vi "ABB Configure temperatures.vi"() -> ()   [LabVIEW 2017]
uses:
  TC Type.ctl
  RTD Type.ctl
  Temp error msg.ctl
  ABB global.vi
panel:
  in  "Temp error":T1="Error: Temperature measurement "
  in  "RTD Type":T2 items=["PT100 3W", "PT100 4W", "PT1000 3W", "PT1000 4W"]
  out "Readings":dbl[](array[numeric])
  in  "Set RTD name":bool
  in  "thermocouple type":i32(ring)=10072 items=["J"=10072, "K"=10073, "N"=10077, "R"=10082, "S"=10085, "T"=10086, "B"=10047, "E"=10055]
  in  "Thermocouple Type":T3 items=["J", "K", "N", "R", "S", "T", "B", "E"]
  in  "RTDs":i32(listbox)
  in  "Enter Name":T4
  in  "Edit names":T5
  in  "Set TC name":bool
  in  "Thermocouples":i32(listbox)
  in  "Exit":bool
  in  "Temperature names":i32(listbox)
  # "Configure Temperature Measurements"
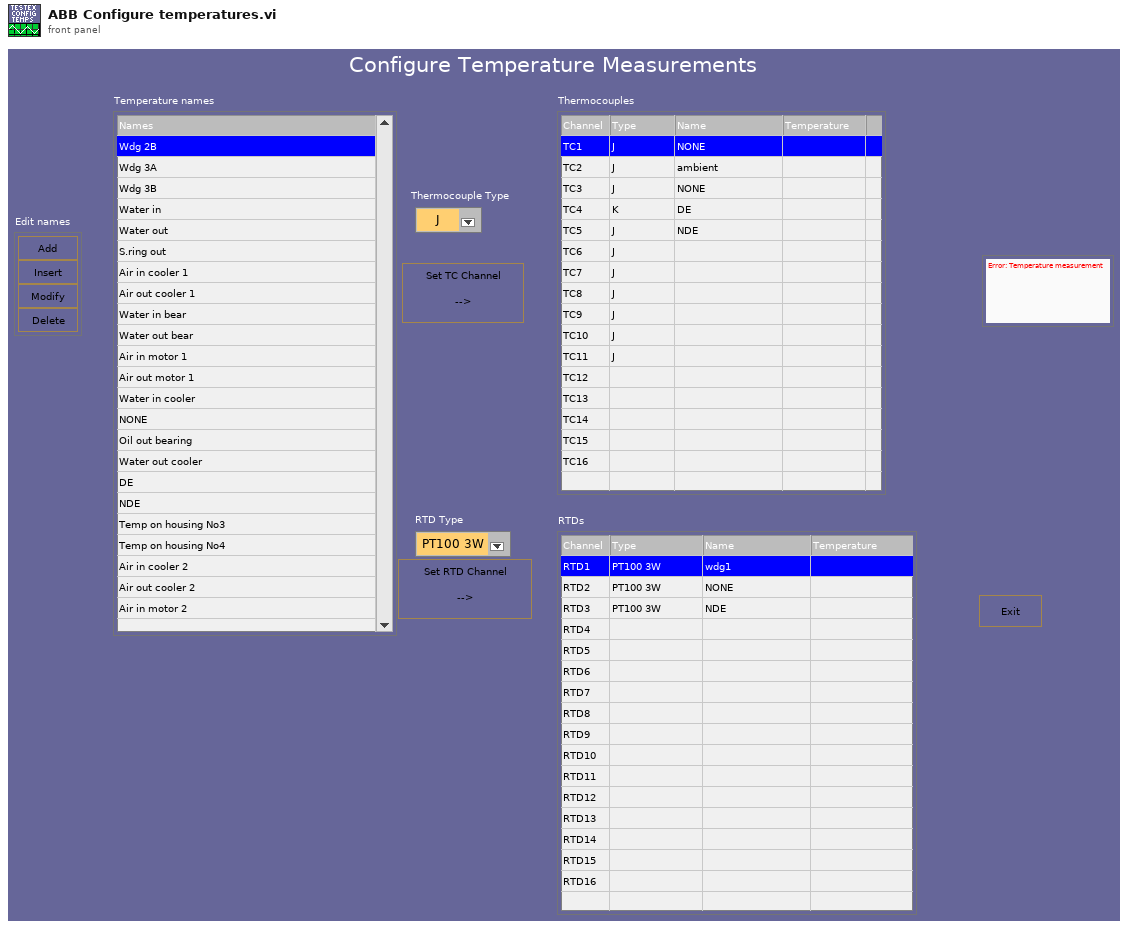
[diagram p1: front panel]
types:
  T1 = typedef "Temp error msg.ctl" = string
  T2 = typedef "RTD Type.ctl" = u16
  T3 = typedef "TC Type.ctl" = u16
  T4 = cluster{"Name":string, "Enter":bool, "Cancel":bool}
  T5 = cluster{"Add":bool, "Insert":bool, "Modify":bool, "Delete":bool}
  T6 = cluster{"Integer":i32, "Dbl":dbl, "String":string, "Boolean":bool}
  T7 = cluster{"Simulate Norma":bool, "Norma 5000 Address":u8, "WebDaq IP Address":string, "Simulate cDAQ":bool}
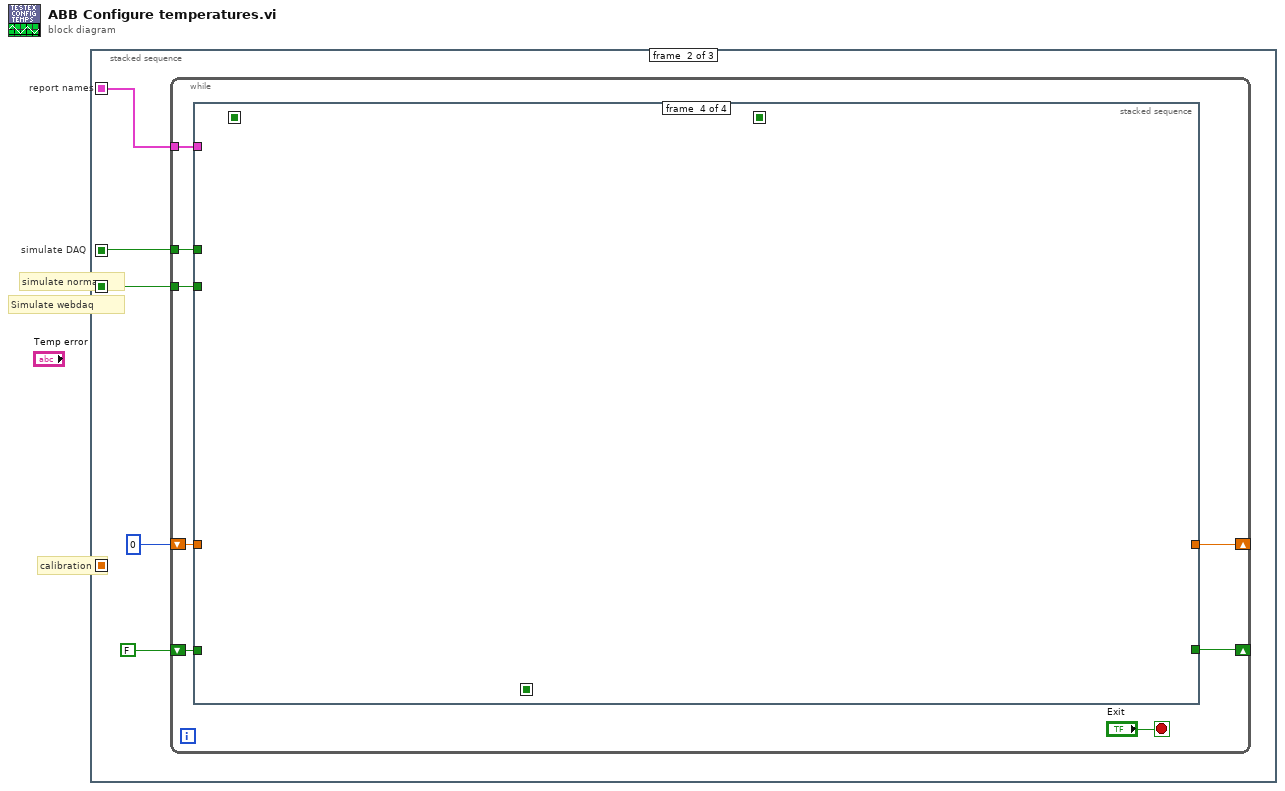
[diagram p0: block diagram]
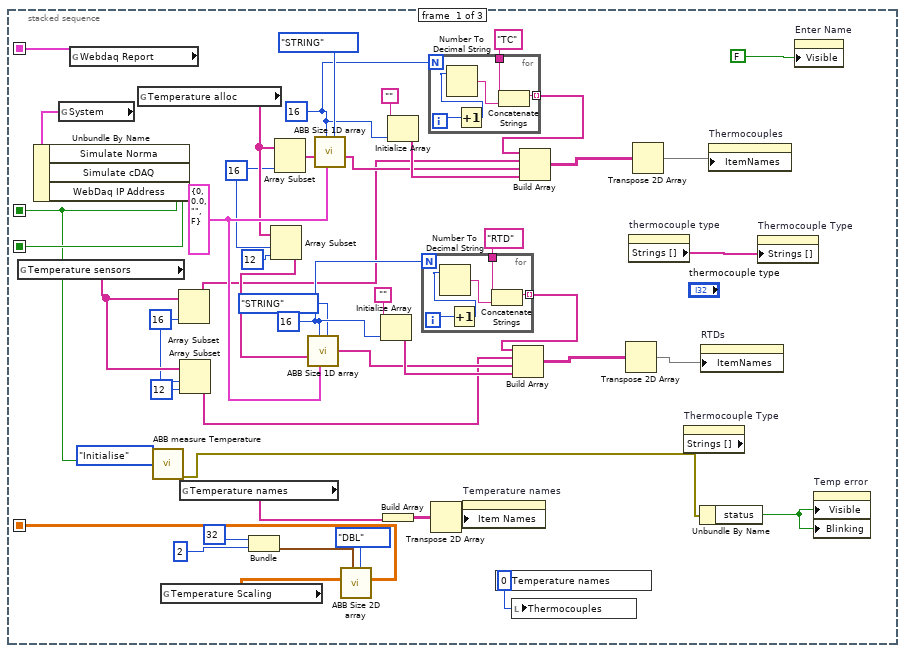
[diagram p2: hidden frame]
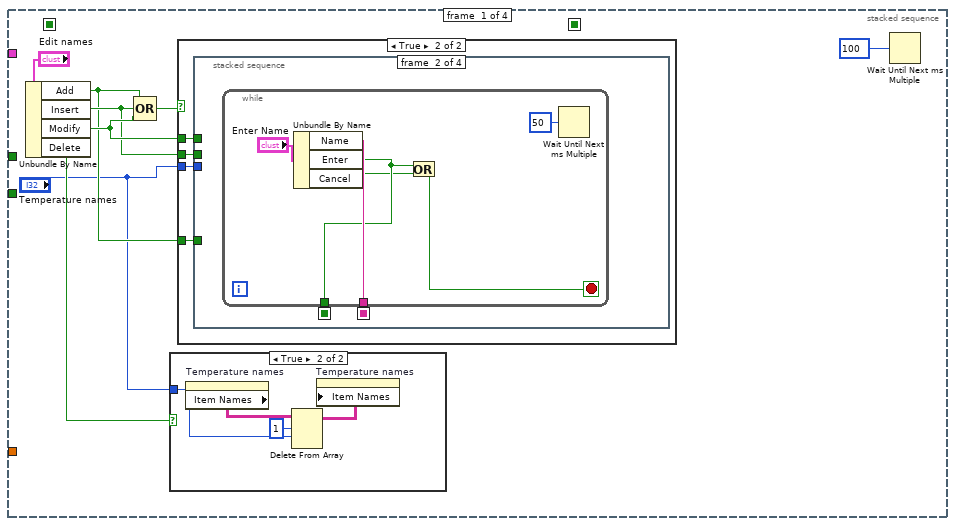
[diagram p3: hidden frame]
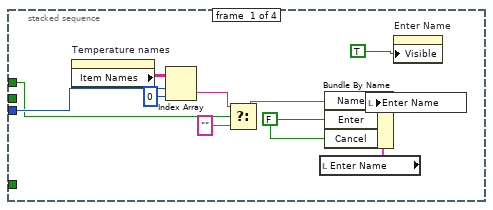
[diagram p6: hidden frame]
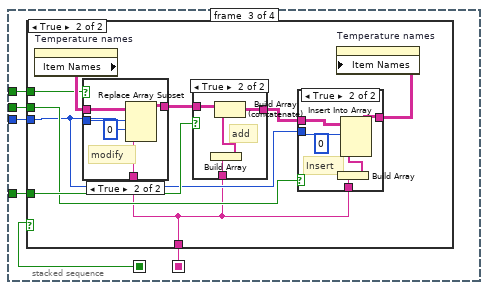
[diagram p7: hidden frame]
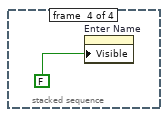
[diagram p12: hidden frame]
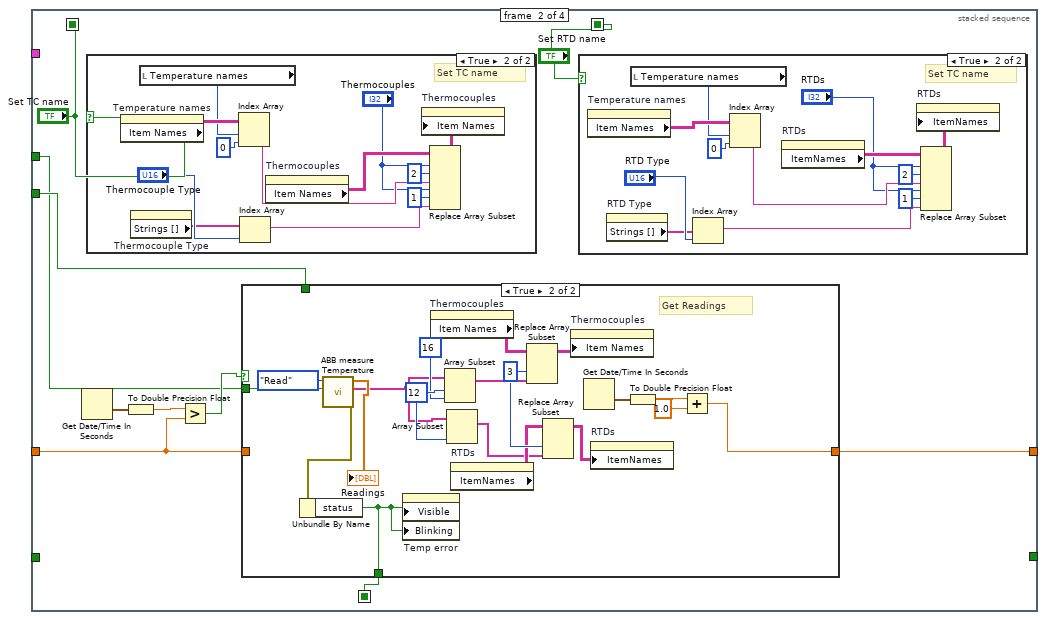
[diagram p13: hidden frame]
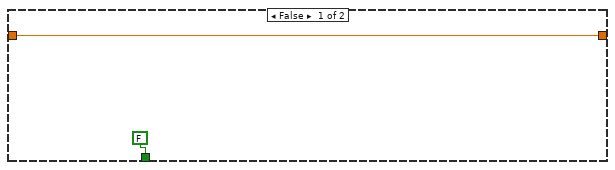
[diagram p15: hidden frame]
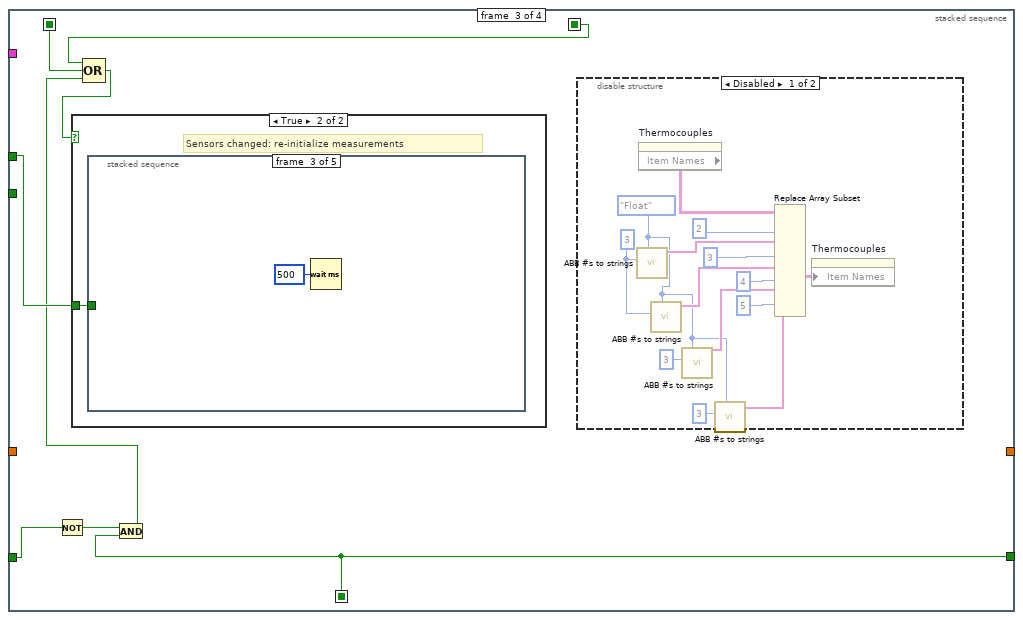
[diagram p17: hidden frame]
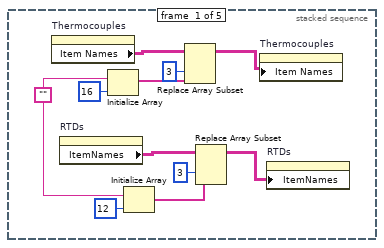
[diagram p20: hidden frame]
diagram:
  # "simulate DAQ"
  # "report names"
  # "Simulate webdaq"
  # "calibration"
  # "simulate norma"
  n1 = stacked-sequence {
    seq-local: [w41 _ _] -> [_ w62 _]
    seq-local: [w35 _ _] -> [_ _ _]
    seq-local: [w33 _ _] -> [_ w61 _]
    seq-local: [w3 _ _] -> [_ w60 w235]
    frame #0 {
      w5 = 16 ("length")
      w17 = 16 ("length")
      w26 = 16 ("Size")
      w20 = T6 {"Integer"=0, "Dbl"=0.0, "String"="", "Boolean"=FALSE} ("Default")
      w43 = 0 ("Temperature names")
      w30 = 16 ("Size")
      n2 = global read "ABB global.vi" "Temperature sensors"() -> (w6:string[])
      n3 = global read "ABB global.vi" "System"() -> (w42:T7)
      n4 = Unbundle By Name(w42) -> ("Simulate Norma"=w41:bool, "Simulate cDAQ"=w3:bool)  [unwired: 1 out]
      n5 = global read "ABB global.vi" "Webdaq Report"() -> (w33:cluster{"Report":string, "Interval":string})
      n6 = global read "ABB global.vi" "Temperature alloc"() -> (w18:string[])
      n7 = call "ABB measure Temperature.vi"("Simulate"=w3, "Mode"=enum16{"Initialise", "Read", "Close"}."Initialise") -> ("error out"=w2:errorcluster)  [unwired: 7 in, 2 out]
      n8 = global read "ABB global.vi" "Temperature Scaling"() -> (w40:dbl[][])
      n9 = Array Subset(array=w6, length=w5) -> (w8:string[])  [unwired: 1 in]
      n10 = Array Subset(array=w6, index=w5, length=12) -> (w4:string[])
      n11 = global read "ABB global.vi" "Temperature names"() -> (w44:string[])
      n12 = Bundle(32, 2) -> (w36:cluster{i32, i32})  [unwired: 1 in]
      n13 = Array Subset(array=w18, index=w17, length=12) -> (w15:string[])
      n14 = Array Subset(array=w18, length=w17) -> (w19:string[])  [unwired: 1 in]
      n15 = call "ABB Size 1D array.vi"("Type"=enum16{"Integer", "DBL", "STRING", "BOOLEAN"}."STRING", "Default"=w20, "Size"=w26, "String Array in"=w15) -> ("String Array out"=w9:string[])  [unwired: 4 in, 3 out]
      n16 = call "ABB Size 1D array.vi"("Type"=enum16{"Integer", "DBL", "STRING", "BOOLEAN"}."STRING", "Default"=w20, "Size"=w30, "String Array in"=w19) -> ("String Array out"=w10:string[])  [unwired: 4 in, 3 out]
      n17 = call "ABB Size 2D array.vi"("Type"=enum16{"Integer", "DBL", "STRING", "BOOLEAN"}."DBL", "Size"=w36, "DBL Array In"=w40) -> ("DBL Array out"=w35:dbl[][])  [unwired: 5 in, 3 out]
      n18 = Initialize Array("", w26) -> (w25:string[])
      n19 = Build Array(w44) -> (w46:string[][])
      n20 = Initialize Array("", w30) -> (w31:string[])
      n21 = for {
        N: w26 -> [_]
        tunnel: "RTD" -> [w53]
        tunnel: [w49] -> w27 mode=indexing
        i -> [w52]
        n22 = Increment(x=w52) -> (x+1=w51:i32)
        n23 = Number To Decimal String(number=w51) -> (decimal integer string=w50:string)  [unwired: 1 in]
        n24 = Concatenate Strings(w53, w50) -> (w49:string)
      }
      n25 = for {
        N: w30 -> [_]
        tunnel: "TC" -> [w58]
        tunnel: [w54] -> w28 mode=indexing
        i -> [w57]
        n26 = Increment(x=w57) -> (x+1=w56:i32)
        n27 = Number To Decimal String(number=w56) -> (decimal integer string=w55:string)  [unwired: 1 in]
        n28 = Concatenate Strings(w58, w55) -> (w54:string)
      }
      n29 = Transpose 2D Array(2D array=w46) -> (transposed array=w45:string[][])
      n30 = property on="Temperature names" class="MCListbox (strict)"("Item Names"=w45) -> ()  [unwired: 2 in, 2 out]
      n31 = local write "Temperature names"(w43) -> ()
      n32 = local write "Thermocouples"(w43) -> ()
      n33 = Build Array(w27, w4, w9, w25) -> (w23:string[][])
      n34 = Build Array(w28, w8, w10, w31) -> (w47:string[][])
      n35 = Transpose 2D Array(2D array=w23) -> (transposed array=w13:string[][])
      n36 = property on="thermocouple type" class="Ring (strict)"() -> ("Strings []"=w12:string[])  [unwired: 2 in, 2 out]
      n37 = Transpose 2D Array(2D array=w47) -> (transposed array=w14:string[][])
      n38 = property on="Thermocouple Type" class="Ring (strict)" props=["Strings []"]() -> ()  [unwired: 2 in, 3 out]
      n39 = Unbundle By Name(w2) -> ("status"=w1:bool)
      n40 = property on="RTDs" class="MCListbox (strict)"("ItemNames"=w13) -> ()  [unwired: 2 in, 2 out]
      n41 = property on="Thermocouples" class="MCListbox (strict)"("ItemNames"=w14) -> ()  [unwired: 2 in, 2 out]
      n42 = property on="Thermocouple Type" class="Ring (strict)"("Strings []"=w12) -> ()  [unwired: 2 in, 2 out]
      n43 = property on="Enter Name" class="Clust (strict)"("Visible"=FALSE) -> ()  [unwired: 2 in, 2 out]
      n44 = property on="Temp error" class="Str (strict)"("Visible"=w1, "Blinking"=w1) -> ()  [unwired: 2 in, 2 out]
    }
    frame #1 {
      n45 = while {
        shift-right: [w69] -> _
        shift-left: 0 -> [w70]
        tunnel: w62 -> [w68]
        tunnel: w61 -> [w67]
        tunnel: w60 -> [w66]
        shift-right: [w65] -> _
        shift-left: FALSE ("status") -> [w64]
        stop <- "Exit" stop-if-true
        n46 = stacked-sequence {
          seq-local: [_ "Set TC name" _ _] -> [_ _ w202 _]
          seq-local: [_ "Set RTD name" _ _] -> [_ _ w201 _]
          seq-local: [_ w140 _ _] -> [_ _ w198 _]
          tunnel: w70 -> [_ w147 _ _]
          tunnel: [_ w149 _ _] -> w69
          tunnel: w68 -> [_ w144 _ _]
          tunnel: w67 -> [_ _ _ _]
          tunnel: w66 -> [_ w141 w199 _]
          tunnel: [_ _ w198 _] -> w65
          tunnel: w64 -> [_ _ w197 _]
          frame #0 {
            n47 = Unbundle By Name("Edit names") -> ("Add"=w74:bool, "Insert"=w75:bool, "Modify"=w76:bool, "Delete"=w73:bool)
            n48 = Compound Arithmetic op=OR(w74, w75, w76) -> (w77:bool)
            n49 = case shown="True" w73 {
              tunnel: "Temperature names" -> [_ w83]
              frame False {
              }
              frame True {
                n50 = property on="Temperature names" class="MCListbox (strict)"() -> ("Item Names"=w82:string[][])  [unwired: 2 in, 2 out]
                n51 = Delete From Array(array=w82, length=1, index (row)=w83) -> (array with subset deleted=w81:string[][])  [unwired: 1 in, 1 out]
                n52 = property on="Temperature names" class="MCListbox (strict)"("Item Names"=w81) -> ()  [unwired: 2 in, 2 out]
              }
            }
            n53 = case shown="True" w77 {
              tunnel: w76 -> [_ w87]
              tunnel: "Temperature names" -> [_ w86]
              tunnel: w75 -> [_ w85]
              tunnel: w74 -> [_ w84]
              frame False {
              }
              frame True {
                n54 = stacked-sequence {
                  seq-local: [_ w100 _ _] -> [_ _ w108 _]
                  seq-local: [_ w99 _ _] -> [_ _ w109 _]
                  tunnel: w87 -> [w95 _ w112 _]
                  tunnel: w86 -> [w98 _ w110 _]
                  tunnel: w85 -> [_ _ w111 _]
                  tunnel: w84 -> [_ _ w107 _]
                  frame #0 {
                    w89 = FALSE ("Enter")
                    n55 = property on="Temperature names" class="MCListbox (strict)"() -> ("Item Names"=w97:string[][])  [unwired: 2 in, 2 out]
                    n56 = Index Array(array=w97, index (row)=w98, index (col)=0 ("disabled index (col)")) -> (element=w94:string)
                    n57 = Select(t=w94, s=w95, f="") -> (s? t:f=w90:string)
                    n58 = local read "Enter Name"() -> (w92:T4)
                    n59 = Bundle By Name(cluster=w92, "Name"=w90, "Enter"=w89, "Cancel"=w89) -> (w91:T4)
                    n60 = local write "Enter Name"(w91) -> ()
                    n61 = property on="Enter Name" class="Clust (strict)"("Visible"=TRUE) -> ()  [unwired: 2 in, 2 out]
                  }
                  frame #1 {
                    n62 = while {
                      tunnel: [w104] -> w100
                      tunnel: [w103] -> w99
                      stop <- w101 stop-if-true
                      n63 = Unbundle By Name("Enter Name") -> ("Name"=w104:string, "Enter"=w103:bool, "Cancel"=w102:bool)
                      n64 = Or(x=w103, y=w102) -> (x .or. y?=w101:bool)
                      n65 = Wait Until Next ms Multiple(millisecond multiple=u32 50) -> ()  [unwired: 1 out]
                    }
                  }
                  frame #2 {
                    n66 = case shown="True" w109 {
                      tunnel: w112 -> [_ w120]
                      tunnel: w111 -> [_ w116]
                      tunnel: w110 -> [_ w115]
                      tunnel: w108 -> [_ w113]
                      tunnel: w107 -> [_ w117]
                      frame False {
                      }
                      frame True {
                        n67 = property on="Temperature names" class="MCListbox (strict)"() -> ("Item Names"=w121:string[][])  [unwired: 2 in, 2 out]
                        n68 = case shown="True" w120 {
                          tunnel: w121 -> [w133 w138]
                          tunnel: [w133 w137] -> w119
                          tunnel: w115 -> [_ w136]
                          tunnel: w113 -> [_ w134]
                          frame False {
                          }
                          frame True {
                            # "modify"
                            n69 = Replace Array Subset(array=w138, new element=w134, index (row)=w136, index (col)=0 ("disabled index (col)")) -> (w137:string[][])
                          }
                        }
                        n70 = case shown="True" w117 {
                          tunnel: w119 -> [w128 w132]
                          tunnel: w113 -> [_ w131]
                          tunnel: [w128 w129] -> w118
                          frame False {
                          }
                          frame True {
                            # "add"
                            n71 = Build Array(w131) -> (w130:string[])
                            n72 = Build Array (concatenate)(w132, w130) -> (w129:string[][])
                          }
                        }
                        n73 = case shown="True" w116 {
                          tunnel: w118 -> [w122 w127]
                          tunnel: [w122 w126] -> w114
                          tunnel: w115 -> [_ w125]
                          tunnel: w113 -> [_ w124]
                          frame False {
                          }
                          frame True {
                            (unwired) 0 ("disabled index (col)")
                            # "Insert"
                            n74 = Build Array(w124) -> (w123:string[])
                            n75 = Insert Into Array(array=w127, index (row)=w125, new element=w123) -> (w126:string[][])  [unwired: 1 in]
                          }
                        }
                        n76 = property on="Temperature names" class="MCListbox (strict)"("Item Names"=w114) -> ()  [unwired: 2 in, 2 out]
                      }
                    }
                  }
                  frame #3 {
                    n77 = property on="Enter Name" class="Clust (strict)"("Visible"=FALSE) -> ()  [unwired: 2 in, 2 out]
                  }
                }
              }
            }
            n78 = Wait Until Next ms Multiple(millisecond multiple=u32 100) -> ()  [unwired: 1 out]
          }
          frame #1 {
            n79 = Get Date/Time In Seconds() -> (seconds since 1Jan1904=w148:timestamp)
            n80 = case shown="True" "Set TC name" {
              frame False {
              }
              frame True {
                # "Set TC name"
                n81 = property on="Temperature names" class="MCListbox (strict)"() -> ("Item Names"=w194:string[][])  [unwired: 2 in, 2 out]
                n82 = property on="Thermocouple Type" class="Ring (strict)"() -> ("Strings []"=w184:string[])  [unwired: 2 in, 2 out]
                n83 = local read "Temperature names"() -> (w193:i32)
                n84 = Index Array(array=w194, index (row)=w193, index (col)=0 ("disabled index (col)")) -> (element=w189:string)
                n85 = Index Array(array=w184, index="Thermocouple Type") -> (element=w185:string)
                n86 = property on="Thermocouples" class="MCListbox (strict)"() -> ("Item Names"=w191:string[][])  [unwired: 2 in, 2 out]
                n87 = Replace Array Subset(array=w191, new element #1=w189, index (row) #1="Thermocouples", index (col) #1=2 ("disabled index (col)"), new element #2=w185, index (row) #2="Thermocouples", index (col) #2=1 ("disabled index (col)")) -> (w188:string[][])
                n88 = property on="Thermocouples" class="MCListbox (strict)"("Item Names"=w188) -> ()  [unwired: 2 in, 2 out]
              }
            }
            n89 = To Double Precision Float(number=w148) -> (double precision float=w145:dbl)
            n90 = Greater?(x=w145, y=w147) -> (0:w146:bool)
            n91 = case shown="True" w146 {
              tunnel: w147 -> [w163 _]
              tunnel: [w163 w177] -> w149
              tunnel: w144 -> [_ _]
              tunnel: w141 -> [_ w167]
              tunnel: [FALSE ("status") w165] -> w140
              frame False {
              }
              frame True {
                w174 = 12 ("index")
                w173 = 3 ("disabled index (col)")
                # "Get Readings"
                n92 = call "ABB measure Temperature.vi"("Simulate"=w167, "Mode"=enum16{"Initialise", "Read", "Close"}."Read") -> ("error out"=w166:errorcluster, "Reading strings"=w164:string[], "Readings"=→"Readings":dbl[])  [unwired: 7 in]
                n93 = Unbundle By Name(w166) -> ("status"=w165:bool)
                n94 = property on="Temp error" class="Str (strict)"("Visible"=w165, "Blinking"=w165) -> ()  [unwired: 2 in, 2 out]
                n95 = property on="Thermocouples" class="MCListbox (strict)"() -> ("Item Names"=w182:string[][])  [unwired: 2 in, 2 out]
                n96 = Array Subset(array=w164, index=w174, length=16) -> (w175:string[])
                n97 = Array Subset(array=w164, length=w174) -> (w170:string[])  [unwired: 1 in]
                n98 = property on="RTDs" class="MCListbox (strict)"() -> ("ItemNames"=w172:string[][])  [unwired: 2 in, 2 out]
                n99 = Replace Array Subset(array=w182, new element=w175, index (col)=w173) -> (w181:string[][])  [unwired: 1 in]
                n100 = Replace Array Subset(array=w172, new element=w170, index (col)=w173) -> (w171:string[][])  [unwired: 1 in]
                n101 = property on="Thermocouples" class="MCListbox (strict)"("Item Names"=w181) -> ()  [unwired: 2 in, 2 out]
                n102 = Get Date/Time In Seconds() -> (seconds since 1Jan1904=w179:timestamp)
                n103 = property on="RTDs" class="MCListbox (strict)"("ItemNames"=w171) -> ()  [unwired: 2 in, 2 out]
                n104 = To Double Precision Float(number=w179) -> (double precision float=w180:dbl)
                n105 = Add(x=w180, y=1.0) -> (x+y=w177:dbl)
              }
            }
            n106 = case shown="True" "Set RTD name" {
              frame False {
              }
              frame True {
                # "Set TC name"
                n107 = property on="Temperature names" class="MCListbox (strict)"() -> ("Item Names"=w161:string[][])  [unwired: 2 in, 2 out]
                n108 = property on="RTD Type" class="Ring (strict)"() -> ("Strings []"=w152:string[])  [unwired: 2 in, 2 out]
                n109 = local read "Temperature names"() -> (w160:i32)
                n110 = Index Array(array=w152, index="RTD Type") -> (element=w155:string)
                n111 = Index Array(array=w161, index (row)=w160, index (col)=0 ("disabled index (col)")) -> (element=w157:string)
                n112 = property on="RTDs" class="MCListbox (strict)"() -> ("ItemNames"=w151:string[][])  [unwired: 2 in, 2 out]
                n113 = Replace Array Subset(array=w151, new element #1=w157, index (row) #1="RTDs", index (col) #1=2 ("disabled index (col)"), new element #2=w155, index (row) #2="RTDs", index (col) #2=1 ("disabled index (col)")) -> (w154:string[][])
                n114 = property on="RTDs" class="MCListbox (strict)"("ItemNames"=w154) -> ()  [unwired: 2 in, 2 out]
              }
            }
          }
          frame #2 {
            n115 = Not(x=w197) -> (.not. x?=w196:bool)
            n116 = And(x=w196, y=w198) -> (x .and. y?=w195:bool)
            n117 = Compound Arithmetic op=OR(w201, w202, w195) -> (w200:bool)
            n118 = case shown="True" w200 {
              tunnel: w199 -> [_ w217]
              frame False {
              }
              frame True {
                # "Sensors changed: re-initialize measurements"
                n119 = stacked-sequence {
                  tunnel: w217 -> [_ w229 _ w232 _]
                  frame #0 {
                    w220 = ""
                    n120 = property on="Thermocouples" class="MCListbox (strict)"() -> ("Item Names"=w228:string[][])  [unwired: 2 in, 2 out]
                    n121 = property on="RTDs" class="MCListbox (strict)"() -> ("ItemNames"=w222:string[][])  [unwired: 2 in, 2 out]
                    n122 = Initialize Array(w220, 16 ("dimension size")) -> (w223:string[])
                    n123 = Initialize Array(w220, 12 ("dimension size")) -> (w219:string[])
                    n124 = Replace Array Subset(array=w228, new element=w223, index (col)=3 ("disabled index (col)")) -> (w226:string[][])  [unwired: 1 in]
                    n125 = Replace Array Subset(array=w222, new element=w219, index (col)=3 ("disabled index (col)")) -> (w218:string[][])  [unwired: 1 in]
                    n126 = property on="Thermocouples" class="MCListbox (strict)"("Item Names"=w226) -> ()  [unwired: 2 in, 2 out]
                    n127 = property on="RTDs" class="MCListbox (strict)"("ItemNames"=w218) -> ()  [unwired: 2 in, 2 out]
                  }
                  frame #1 {
                    n128 = call "ABB measure Temperature.vi"("Simulate"=w229, "Mode"=enum16{"Initialise", "Read", "Close"}."Close") -> ()  [unwired: 7 in, 3 out]
                  }
                  frame #2 {
                    n129 = Wait (ms)(milliseconds to wait=u32 500) -> ()  [unwired: 1 out]
                  }
                  frame #3 {
                    n130 = call "ABB measure Temperature.vi"("Simulate"=w232, "Mode"=enum16{"Initialise", "Read", "Close"}."Initialise") -> ()  [unwired: 7 in, 3 out]
                  }
                  frame #4 {
                    n131 = Wait (ms)(milliseconds to wait=u32 500) -> ()  [unwired: 1 out]
                  }
                }
              }
            }
            n132 = disable-structure shown="Disabled" {
              frame Disabled {
                w213 = 3 ("Precision")
                w208 = enum16{"Float", "Relative time HH:MM"}."Float" ("# type")
                n133 = call "ABB #s to strings.vi"("# type"=w208, "Precision"=w213) -> ("Strings out"=w215:string[])  [unwired: 9 in]
                n134 = property on="Thermocouples" class="MCListbox (strict)"() -> ("Item Names"=w216:string[][])  [unwired: 2 in, 2 out]
                n135 = call "ABB #s to strings.vi"("# type"=w208, "Precision"=w213) -> ("Strings out"=w212:string[])  [unwired: 9 in]
                n136 = call "ABB #s to strings.vi"("# type"=w208, "Precision"=3) -> ("Strings out"=w211:string[])  [unwired: 9 in]
                n137 = call "ABB #s to strings.vi"("# type"=w208, "Precision"=3) -> ("Strings out"=w207:string[])  [unwired: 9 in]
                n138 = Replace Array Subset(array=w216, new element #1=w215, index (col) #1=2 ("disabled index (col)"), new element #2=w212, index (col) #2=3 ("index (col)"), new element #3=w211, index (col) #3=4 ("index (col)"), new element #4=w207, index (col) #4=5 ("index (col)")) -> (w204:string[][])  [unwired: 4 in]
                n139 = property on="Thermocouples" class="MCListbox (strict)"("Item Names"=w204) -> ()  [unwired: 2 in, 2 out]
              }
              frame Enabled {
              }
            }
          }
          frame #3 {
          }
        }
      }
    }
    frame #2 {
      n140 = Two Button Dialog(message="Save any changes?") -> (T button?=w238:bool)  [unwired: 2 in]
      n141 = call "ABB measure Temperature.vi"("Simulate"=w235, "Mode"=enum16{"Initialise", "Read", "Close"}."Close") -> ()  [unwired: 7 in, 3 out]
      n142 = case shown="True" w238 {
        frame False {
        }
        frame True {
          n143 = stacked-sequence {
            frame #0 {
              n144 = property on="Thermocouples" class="MCListbox (strict)"() -> ("Item Names"=w239:string[][])  [unwired: 2 in, 2 out]
              n145 = property on="RTDs" class="MCListbox (strict)"() -> ("ItemNames"=w240:string[][])  [unwired: 2 in, 2 out]
              n146 = property on="Temperature names" class="MCListbox (strict)"() -> ("Item Names"=w245:string[][])  [unwired: 2 in, 2 out]
              n147 = Build Array (concatenate)(w239, w240) -> (w241:string[][])
              n148 = Index Array(array=w245, index (col)=0 ("disabled index (col)")) -> (element=w244:string[])  [unwired: 1 in]
              n149 = global write "ABB global.vi" "Temperature names"(w244) -> ()
              n150 = Index Array(array=w241, index (col) #1=2 ("disabled index (col)"), index (col) #2=1 ("index (col)")) -> (element #1=w247:string[], element #2=w242:string[])  [unwired: 2 in]
              n151 = global write "ABB global.vi" "Temperature sensors"(w242) -> ()
              n152 = global write "ABB global.vi" "Temperature alloc"(w247) -> ()
            }
            frame #1 {
              n153 = call "ABB Load-Save config.vi"("Mode"=enum16{"LOAD", "SAVE"}."SAVE") -> ()  [unwired: 11 in]
            }
          }
        }
      }
    }
  }
